vi "02Foot.vi"() -> ()   [LabVIEW 2015]
uses:
  <vilib>/Utility/file.llb/Write Delimited Spreadsheet (DBL).vi
  <vilib>/Analysis/NI_AALBase.lvlib
panel:
  out "x*y":dbl
  out "size(s)":i32
  out "floor(x/y)":i32
  out "Histogram Graph":T1(graph)
  out "Waveform Graph":dbl[](graph)
  in  "Array":dbl[](array[numeric])
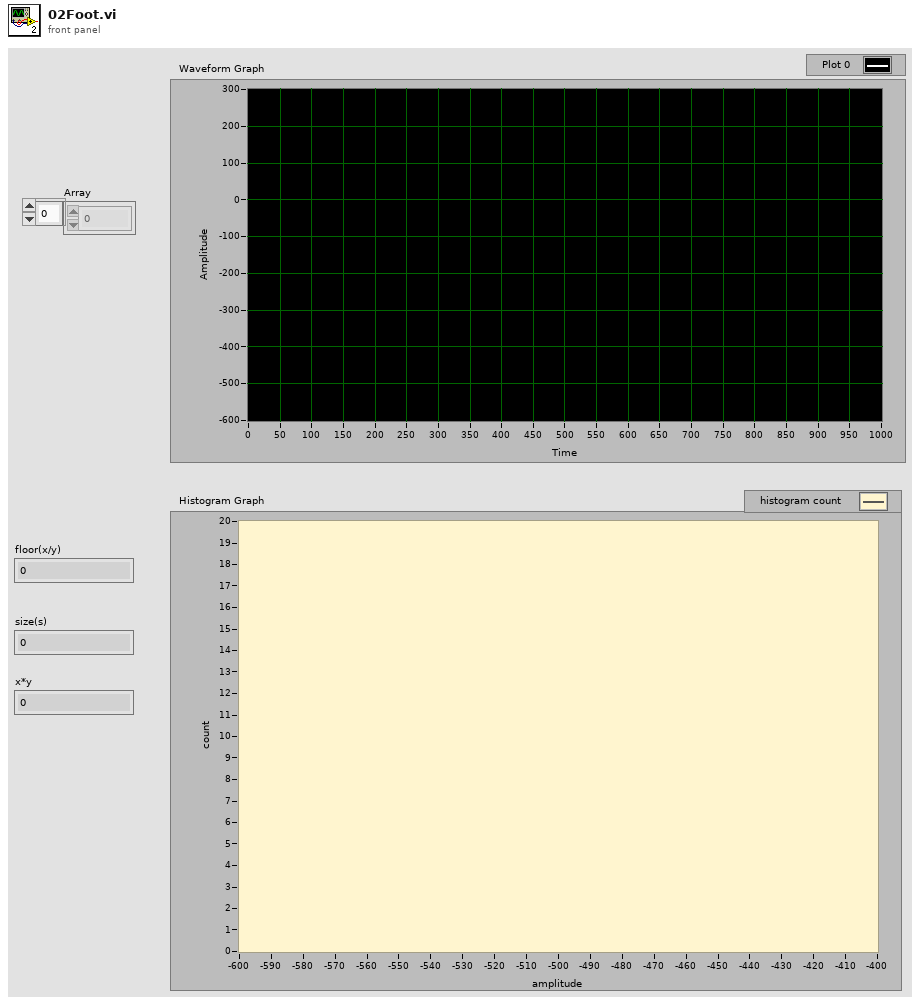
[diagram p1: front panel]
types:
  T1 = cluster{"X Values":dbl[], "Histogram: h(x)":i32[]}
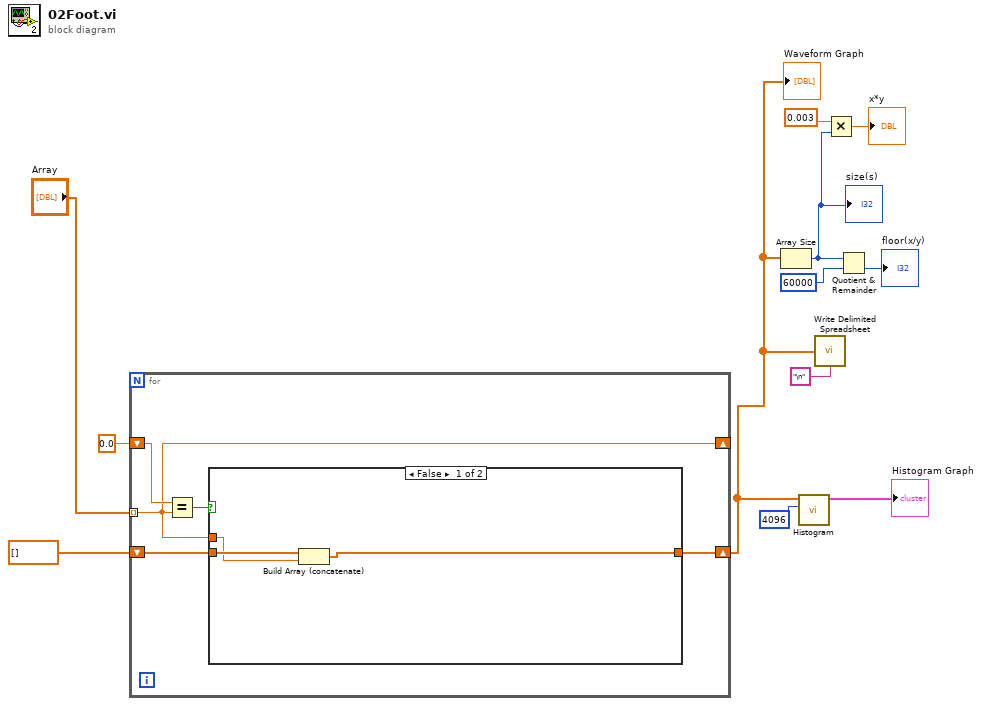
[diagram p0: block diagram]
diagram:
  n1 = for {
    tunnel: "Array" -> [w15] mode=indexing
    shift-right: [w15] -> _
    shift-left: 0.0 -> [w16]
    shift-right: [w13] -> w2
    shift-left: dbl[] [] -> [w14]
    n2 = Equal?(x=w16, y=w15) -> (x = y?=w17:bool)
    n3 = case shown="False" w17 {
      tunnel: w15 -> [w18 _]
      tunnel: w14 -> [w20 w21]
      tunnel: [w19 w21] -> w13
      frame False {
        n4 = Build Array (concatenate)(w20, w18) -> (w19:dbl[])
      }
      frame True {
      }
    }
  }
  "Waveform Graph" <- w2
  n5 = Array Size(array=w2) -> (size(s)=w8:i32)
  "size(s)" <- w8
  n6 = call <vilib>:"Histogram.vi"("intervals"=4096, "X"=w2) -> ("Histogram Graph"=→"Histogram Graph":T1)  [unwired: 6 in, 3 out]
  n7 = call-poly <vilib>:"Write Delimited Spreadsheet.vi"("1D data"=w2, "delimiter (\\t)"="\n" ("delimiter (\\t)")) -> ()  [unwired: 12 in, 2 out]
  n8 = Multiply(x=0.003, y=w8) -> (x*y=→"x*y":dbl)
  n9 = Quotient & Remainder(x=w8, y=60000) -> (floor(x/y)=→"floor(x/y)":i32)  [unwired: 1 out]
